vi "get_next_job.vi"(8 "error in (no error)":errorcluster, 11 "cache path":path) -> (0 "error out":errorcluster, 2 "remaining jobs":i32, 3 "appended path":path)   [LabVIEW 2024, in "Download_Manager.lvlib"]
uses:
  Download_Manager.lvlib
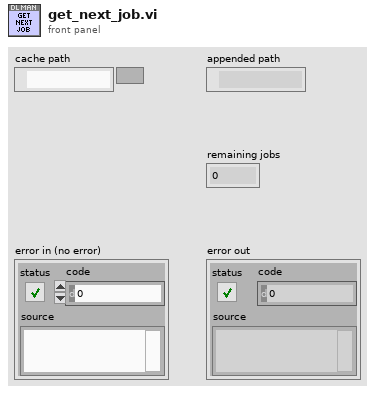
[diagram p1: front panel]
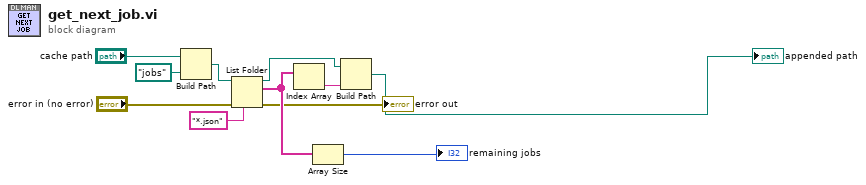
[diagram p0: block diagram]
diagram:
  n1 = Build Path(base path="cache path", name or relative path=path "jobs") -> (appended path=w5:path)
  n2 = List Folder(path=w5, pattern="*.json", error in="error in (no error)") -> (path out=w8:path, filenames=w10:string[], error out=→"error out":errorcluster)  [unwired: 1 in, 1 out]
  n3 = Index Array(array=w10) -> (element=w7:string)  [unwired: 1 in]
  n4 = Array Size(array=w10) -> (size(s)=→"remaining jobs":i32)
  n5 = Build Path(base path=w8, name or relative path=w7) -> (appended path=→"appended path":path)
